vi "MAAP1.vi"() -> ()   [LabVIEW 2016]
doc: "Use this VI to generate and filter noisy signals using low and high pass filters including higher order Butterworth filters.\n\nMuhannad Alghamdi\nCSUSB Physics 350"
uses:
  typedefs/periodic_signal_control.ctl
  <vilib>/ptbypt/NI_PtbyPt.lvlib
panel:
  in  "stop":bool
  in  "Update interval":u32(slide)=20 scale=1.0..1000.0
  in  "Order":enum16{"1st order", "2nd order", "3rd order"}(ring)=enum."3rd order"
  in  "Corner period":dbl(slide)=50.0 scale=1.0..1000.0
  in  "Low pass":bool=TRUE
  in  "Order":enum16{"1st order", "2nd order", "3rd order"}(ring)
  in  "Corner period":dbl(slide)=1.0 scale=1.0..1000.0
  in  "High pass":bool
  in  "White noise":bool
  in  "Amplitude":dbl(slide)=0.2 scale=0.0..1.0
  in  "Signals mode":bool
  in  "Source 2":T1={"Source"=TRUE, "Source type"=TRUE, "Amplitude"=1.0, "Period"=100.0} {"Amplitude" scale=0.0..1.0; "Period" scale=1.0..1000.0}
  in  "Source 1":T1={"Source"=TRUE, "Source type"=TRUE, "Amplitude"=1.0, "Period"=10.0} {"Amplitude" scale=0.0..1.0; "Period" scale=1.0..1000.0}
  out "Waveform chart":cluster{"Signal out":dbl, "output":dbl}(graph)={"Signal out"=-1.939711579865122, "output"=-0.5477725184958412}
  # "Signal Generation and Filtering"
  # "Signal Generation"
  # "Filtering"
  # "High pass"
  # "Low pass"
  # "Source 3"
  # "Muhannad Alghamdi\nProject 1\nPHYS 350"
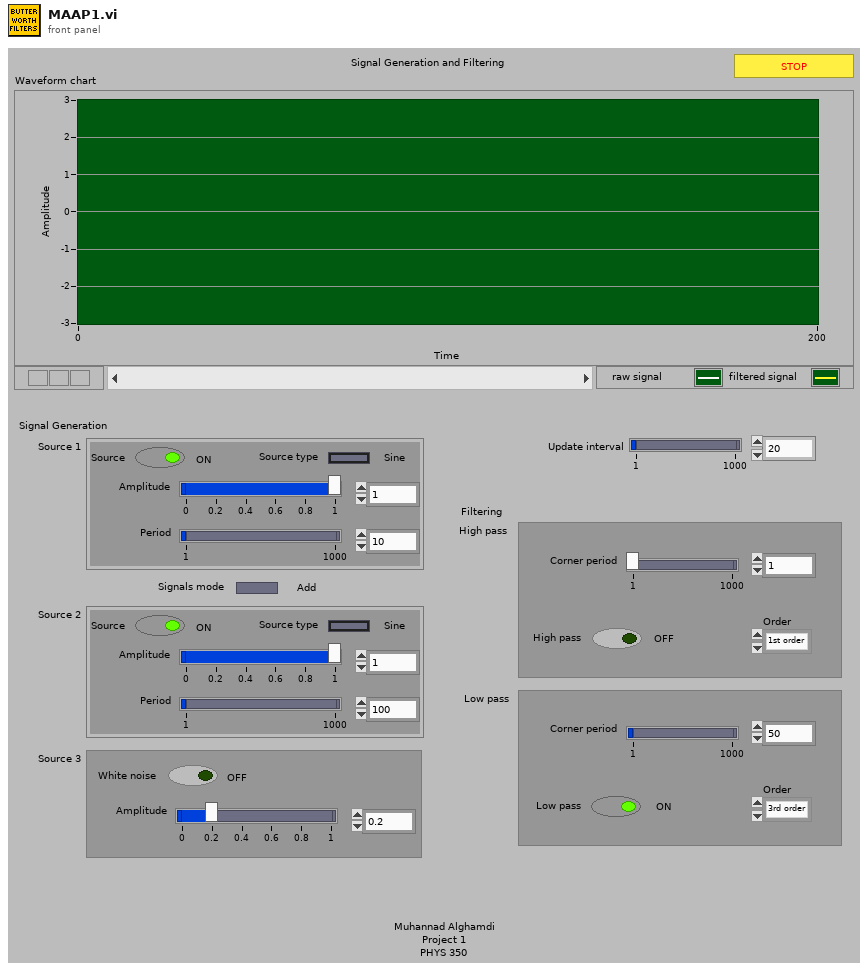
[diagram p1: front panel]
types:
  T1 = typedef "periodic_signal_control.ctl" = cluster{"Source":bool, "Source type":bool, "Amplitude":dbl, "Period":dbl}
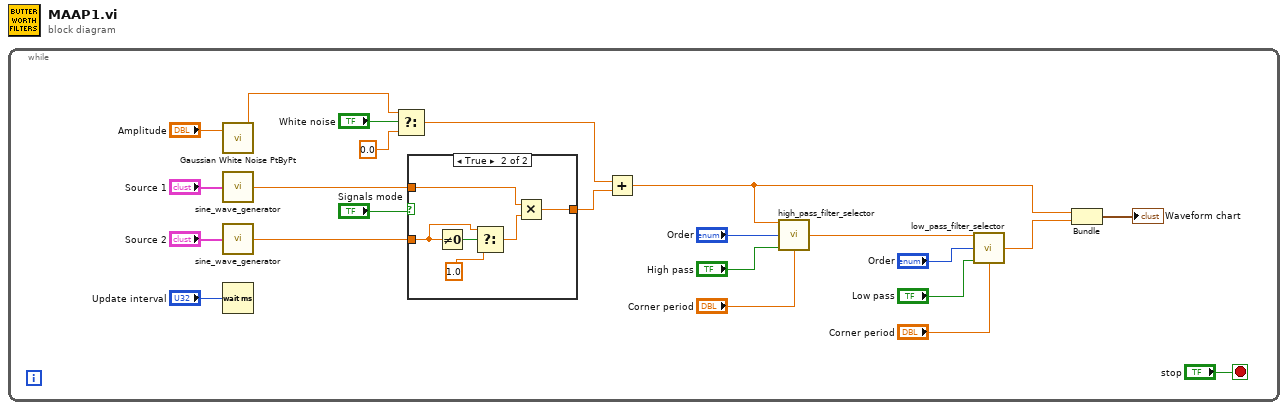
[diagram p0: block diagram]
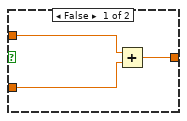
[diagram p2: hidden frame]
diagram:
  n1 = while {
    stop <- "stop" stop-if-true
    n2 = call <vilib>:"Gaussian White Noise PtByPt.vi"("standard deviation"="Amplitude") -> ("Gaussian white noise"=w2:dbl)  [unwired: 2 in]
    n3 = call "sine_wave_generator.vi"("Source"="Source 1") -> ("Output"=w18:dbl)  [unwired: 14 in]
    n4 = call "sine_wave_generator.vi"("Source"="Source 2") -> ("Output"=w16:dbl)  [unwired: 14 in]
    n5 = Wait (ms)(milliseconds to wait="Update interval") -> ()  [unwired: 1 out]
    n6 = Select(t=w2, s="White noise", f=0.0) -> (s? t:f=w3:dbl)
    n7 = case shown="True" "Signals mode" {
      tunnel: w18 -> [w26 w32]
      tunnel: w16 -> [w24 w29]
      tunnel: [w25 w31] -> w17
      frame False {
        n8 = Add(x=w26, y=w24) -> (x+y=w25:dbl)
      }
      frame True {
        n9 = Not Equal To 0?(x=w29) -> (x != 0?=w30:bool)
        n10 = Select(t=w29, s=w30, f=1.0) -> (s? t:f=w27:dbl)
        n11 = Multiply(x=w32, y=w27) -> (x*y=w31:dbl)
      }
    }
    n12 = Add(x=w3, y=w17) -> (x+y=w15:dbl)
    n13 = call "high_pass_filter_selector.vi"("Signal input"=w15, "Order"="Order", "High pass"="High pass", "Corner period"="Corner period") -> ("Signal output"=w11:dbl)  [unwired: 11 in]
    n14 = call "low_pass_filter_selector.vi"("Signal input"=w11, "Order"="Order", "Low pass"="Low pass", "Corner period"="Corner period") -> ("Signal output"=w7:dbl)  [unwired: 11 in]
    n15 = Bundle(w15, "Signal output"=w7) -> (→"Waveform chart":cluster{dbl, "Signal output":dbl})  [unwired: 1 in]
  }
